vi "Actor Core.vi"(8 "error in":errorcluster, 11 "AxisStatus In":refnum<class "AxisStatus.lvclass">) -> (0 "error out":errorcluster, 3 "Actor out":refnum<class "Actor.lvclass">)   [LabVIEW 2020, in "AxisStatus.lvlib" / "AxisStatus.lvclass"]
uses:
  AxisStatus.lvclass
  C:/Program Files (x86)/National Instruments/LabVIEW 2020/vi.lib/gpm_packages/@cs/mva-viewable/Source/IViewable/IViewable/IViewable.lvclass
  <vilib>/ActorFramework/Actor/Actor.lvclass
  Controls/Axis_Control.ctl
  <vilib>/Retry/UI Control Suite/Boolean/System Buttons/Clear Button.ctl
  <vilib>/Retry/UI Control Suite/Boolean/System Buttons/Refresh2 Button.ctl
  <vilib>/Retry/UI Control Suite/Boolean/System Buttons/Stop Button.ctl
  <vilib>/gpm_packages/@cs/mva-viewable/Source/IViewable/IViewable/IViewable.lvclass
  Controls/Controls.lvlib
panel:
  out "IO紧急停止":bool
  out "IO平滑停止":bool
  out "运动状态":bool
  out "伺服使能":bool
  out "运动错误":bool
  out "正限位":bool
  out "负限位":bool
  out "驱动报警":bool
  in  "System Stop Button":bool
  in  "Stop Button":T1
  in  "Refresh Button":T2
  in  "System OK Button":bool
  in  "Clear Button":T3
  out "Axis":T4 caption="轴号"
  out "运动模式":string
  out "规划速度(mm/Sec)":dbl
  out "实际速度(mm/Sec)":dbl
  out "规划位置(mm)":dbl
  out "实际位置(mm)":dbl
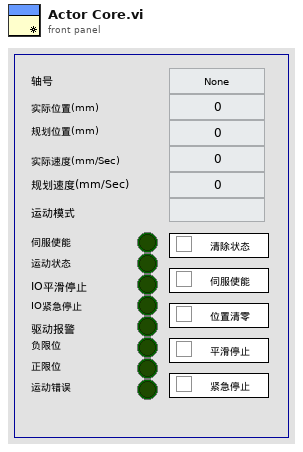
[diagram p1: front panel]
types:
  T1 = typedef "Stop Button.ctl" = bool
  T2 = typedef "Refresh2 Button.ctl" = bool
  T3 = typedef "Clear Button.ctl" = bool
  T4 = typedef "Controls.lvlib/Axis_Control.ctl" = enum16{"None", "1", "2", "3", "4", "5", "6", "7", "8"}
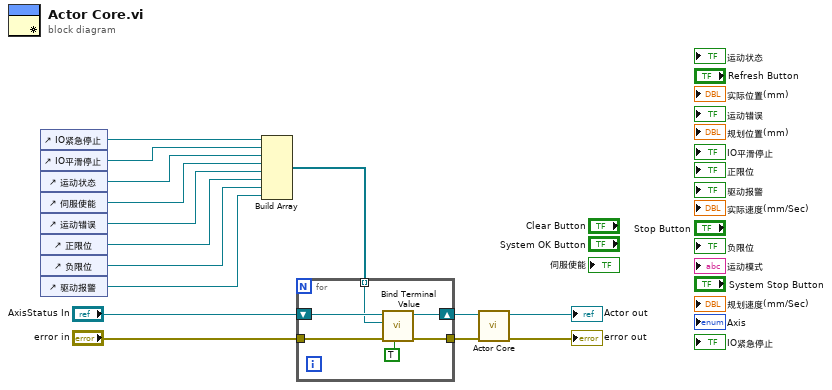
[diagram p0: block diagram]
diagram:
  n1 = control-ref of="IO紧急停止"() -> (w13:refnum<vi>)
  n2 = control-ref of="IO平滑停止"() -> (w12:refnum<vi>)
  n3 = control-ref of="运动状态"() -> (w11:refnum<vi>)
  n4 = control-ref of="伺服使能"() -> (w10:refnum<vi>)
  n5 = control-ref of="运动错误"() -> (w9:refnum<vi>)
  n6 = control-ref of="正限位"() -> (w8:refnum<vi>)
  n7 = control-ref of="负限位"() -> (w7:refnum<vi>)
  n8 = control-ref of="驱动报警"() -> (w6:refnum<vi>)
  n9 = Build Array(w13, w12, w11, w10, w9, w8, w7, w6) -> (w2:refnum<vi>[])
  n10 = for {
    tunnel: [w19] -> w3
    tunnel: w2 -> [w18] mode=indexing
    shift-right: [w20] -> w4
    shift-left: "AxisStatus In" -> [w21]
    tunnel: "error in" -> [w17]
    n11 = call <vilib>:"Bind Terminal Value.vi"("Value Changes Only? (T)"=TRUE, "error in (no error)"=w17, "Ctl Refnum"=w18, "IViewable in"=w21) -> ("error out"=w19:errorcluster, "IViewable out"=w20:refnum<class "AxisStatus.lvclass">)  [unwired: 6 in]
  }
  n12 = call-parent "Actor Core.vi"("error in"=w3, "IViewable In"=w4) -> ("error out"=→"error out":errorcluster, "Actor out"=→"Actor out":refnum<class "Actor.lvclass">)  [unwired: 8 in]
